vi "Current EXE File Path.vi"(8 "error in (no error)":errorcluster) -> (0 "error out":errorcluster, 3 "Current EXE Path":path)   [LabVIEW 2016, in "SLL Application.lvlib"]
doc: "Provides the current EXE file path. \n\nThis will not work in LabVIEW development environment."
uses:
  SLL Application.lvlib
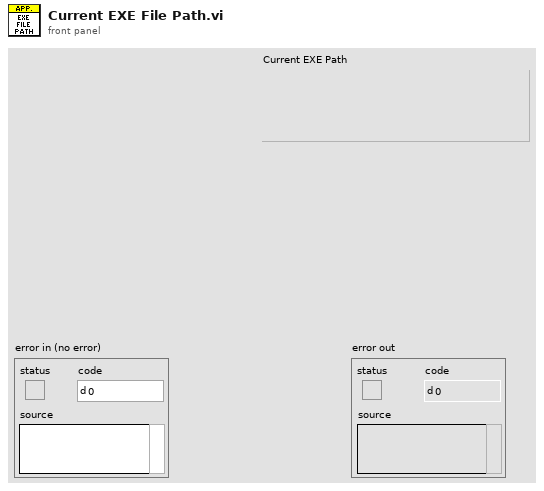
[diagram p1: front panel]
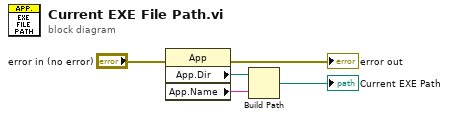
[diagram p0: block diagram]
diagram:
  n1 = property class="App"(error in="error in (no error)") -> (error out=→"error out":errorcluster, "App.Dir"=w4:path, "App.Name"=w5:string)  [unwired: 1 in, 1 out]
  n2 = Build Path(base path=w4, name or relative path=w5) -> (appended path=→"Current EXE Path":path)
